vi "arctan.vi"(1 "x":dbl[](array[numeric])) -> (0 "y":dbl[](array[numeric]))   [LabVIEW 2020]
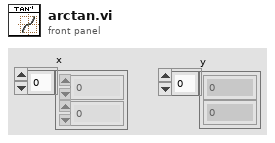
[diagram p1: front panel]
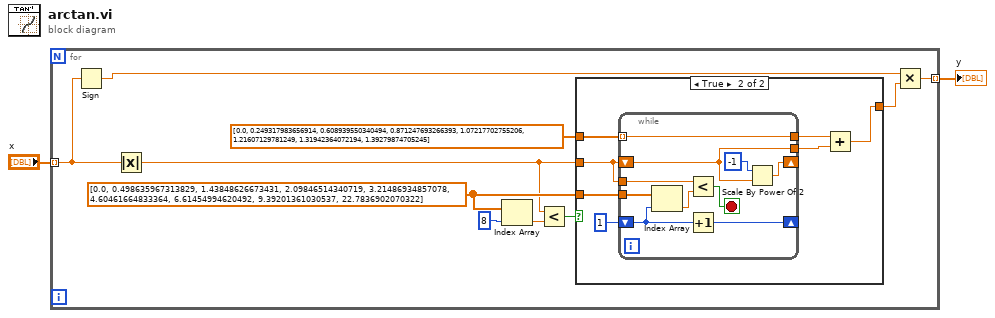
[diagram p0: block diagram]
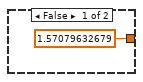
[diagram p2: hidden frame]
diagram:
  n1 = for {
    tunnel: "x" -> [w6] mode=indexing
    tunnel: [w3] -> w1 mode=indexing
    w10 = dbl[] [0.0, 0.498635967313829, 1.43848626673431, 2.09846514340719, 3.21486934857078, 4.60461664833364, 6.61454994620492, 9.39201361030537, 22.7836902070322]
    n2 = Sign(1:w6) -> (0:w5:dbl)
    n3 = Absolute Value(x=w6) -> (abs(x)=w7:dbl)
    n4 = Index Array(array=w10, index=8) -> (element=w11:dbl)
    n5 = Less?(x=w7, y=w11) -> (x < y?=w12:bool)
    n6 = case shown="True" w12 {
      tunnel: w7 -> [_ w19]
      tunnel: [1.57079632679 w18] -> w4
      tunnel: w10 -> [_ w17]
      tunnel: dbl[] [0.0, 0.249317983656914, 0.608939550340494, 0.871247693266393, 1.07217702755206, 1.21607129781249, 1.31942364072194, 1.39279874705245] -> [_ w16]
      frame False {
      }
      frame True {
        n7 = while {
          tunnel: w19 -> [w30]
          shift-right: [w28] -> _
          shift-left: 1 -> [w26]
          shift-right: [w25] -> _
          shift-left: w19 -> [w23]
          tunnel: [w23] -> w15
          tunnel: w17 -> [w22]
          tunnel: [w21] -> w14
          tunnel: w16 -> [w21] mode=indexing
          stop <- w29 stop-if-true
          n8 = Index Array(array=w22, index=w26) -> (element=w27:dbl)
          n9 = Less?(x=w30, y=w27) -> (x < y?=w29:bool)
          n10 = Increment(x=w26) -> (x+1=w28:i32)
          n11 = Scale By Power Of 2(n=-1, x=w23) -> (x*2^n=w25:dbl)
        }
        n12 = Add(x=w14, y=w15) -> (x+y=w18:dbl)
      }
    }
    n13 = Multiply(x=w5, y=w4) -> (x*y=w3:dbl)
  }
  "y" <- w1
